vi "ModeTurret.vi"(1 "Master State":enum16{"Normal", "Climb"}(ring)) -> (0 "Turret Mode":enum16{"Targetting", "Failure Mode", "Climbing"}(ring))   [LabVIEW 2020]
doc: "Determines the appropriate mode for the turret subsystem."
uses:
  driverdata.vi
  drivercommands.vi
  sensordata.vi
  robotoutputs.vi
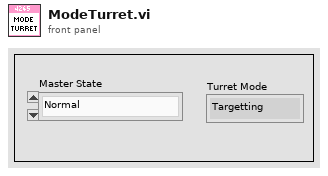
[diagram p1: front panel]
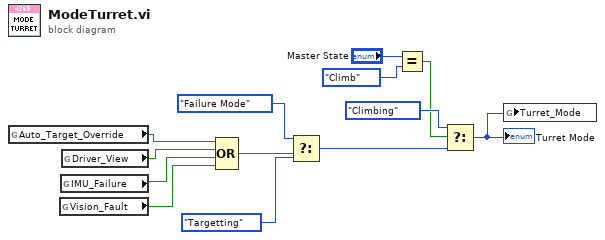
[diagram p0: block diagram]
diagram:
  n1 = global read "driverdata.vi" "Auto_Target_Override"() -> (w5:bool)
  n2 = global read "sensordata.vi" "Vision_Fault"() -> (w2:bool)
  n3 = global read "sensordata.vi" "IMU_Failure"() -> (w3:bool)
  n4 = global read "drivercommands.vi" "Driver_View"() -> (w4:bool)
  n5 = Compound Arithmetic op=OR(w5, w4, w3, w2) -> (w6:bool)
  n6 = Select(t=enum16{"Targetting", "Failure Mode", "Climbing"}."Failure Mode" ("Turret Mode"), s=w6, f=enum16{"Targetting", "Failure Mode", "Climbing"}."Targetting" ("Turret Mode")) -> (s? t:f=w11:enum16{"Targetting", "Failure Mode", "Climbing"})
  n7 = Equal?(x="Master State", y=enum16{"Normal", "Climb"}."Climb" ("Master State")) -> (x = y?=w7:bool)
  n8 = Select(t=enum16{"Targetting", "Failure Mode", "Climbing"}."Climbing" ("Turret Mode"), s=w7, f=w11) -> (s? t:f=w1:enum16{"Targetting", "Failure Mode", "Climbing"})
  "Turret Mode" <- w1
  n9 = global write "robotoutputs.vi" "Turret_Mode"(w1) -> ()
